vi "Process Data.vi"(8 "error in":errorcluster, 11 "Client Manager in":refnum<class "Client Manager.lvclass">) -> (0 "error out":errorcluster, 3 "Client Manager out":refnum<class "Client Manager.lvclass">)   [LabVIEW 2014, in "Client Manager.lvclass"]
uses:
  Client Manager.lvclass
  Topic Child Classes/Launch Client/Launch Client.lvclass
  Architecture/Classes/Topic_class/Topic.lvclass
panel:
  out "Client ID":string
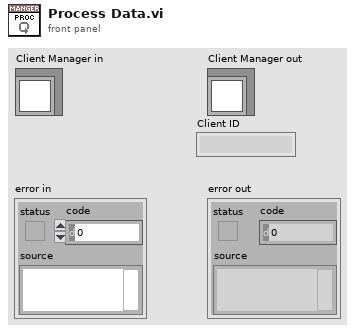
[diagram p1: front panel]
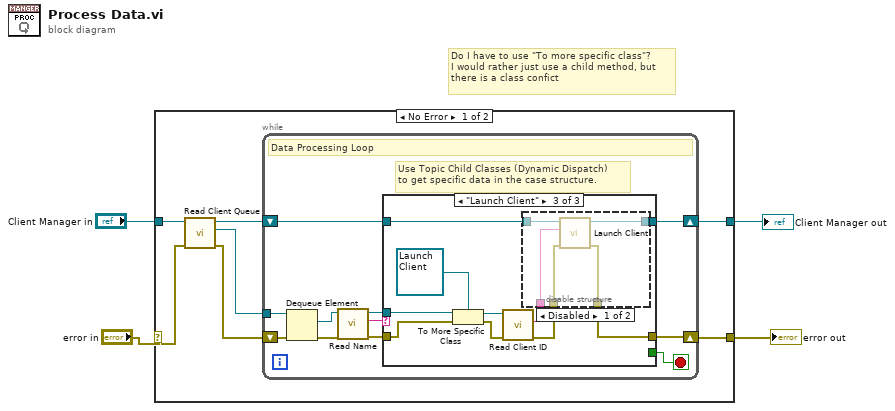
[diagram p0: block diagram]
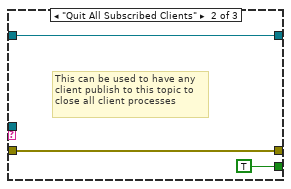
[diagram p3: hidden frame]
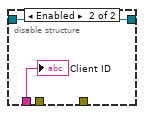
[diagram p4: hidden frame]
diagram:
  # "Do I have to use \"To more specific class\"?\nI would rather just use a child method, but\nthere is a class confict"
  n1 = case shown="No Error" "error in" {
    selector: "error in" -> [w5 w46]
    tunnel: [w6 w46] -> w2
    tunnel: [w8 w45] -> w3
    tunnel: "Client Manager in" -> [w11 w45]
    frame No Error {
      n2 = call-dynamic "Read Client Queue.vi"("error in"=w5, "Client in"=w11) -> ("error out"=w7:errorcluster, "Client Queue"=w10:refnum<queue>, "Client out"=w9:refnum<class "Client Manager.lvclass">)  [unwired: 7 in]
      n3 = while {
        tunnel: w10 -> [w22]
        shift-right: [w14] -> w8
        shift-left: w9 -> [w15]
        shift-right: [w12] -> w6
        shift-left: w7 -> [w13]
        stop <- w16 stop-if-true
        # "Use Topic Child Classes (Dynamic Dispatch)\nto get specific data in the case structure."
        # "Data Processing Loop"
        n4 = Dequeue Element(queue=w22, error in (no error)=w13) -> (element=w20:refnum<class "Topic.lvclass">, error out=w21:errorcluster)  [unwired: 1 in, 2 out]
        n5 = call-dynamic "Read Name.vi"("error in"=w21, "Topic in"=w20) -> ("error out"=w18:errorcluster, "Name"=w19:string, "Topic out"=w17:refnum<class "Topic.lvclass">)  [unwired: 7 in]
        n6 = case shown="\"Launch Client\"" w19 {
          tunnel: [_ TRUE _] -> w16
          tunnel: w18 -> [w24 w26 w32]
          tunnel: [w24 w26 w29] -> w12
          tunnel: w17 -> [_ _ w36]
          tunnel: w15 -> [w23 w25 w37]
          tunnel: [w23 w25 w28] -> w14
          frame Default {
          }
          frame "Quit All Subscribed Clients" {
            # "This can be used to have any\nclient publish to this topic to\nclose all client processes"
          }
          frame "Launch Client" {
            n7 = To More Specific Class(target class=refnum<class "Launch Client.lvclass"> refnum ("Launch Client.lvclass"), reference=w36, error in=w32) -> (specific class reference=w34:refnum<class "Launch Client.lvclass">, error out=w31:errorcluster)
            n8 = call-dynamic "Read Client ID.vi"("error in"=w31, "Launch Client in"=w34) -> ("error out"=w30:errorcluster, "Client ID"=w33:string)  [unwired: 7 in, 1 out]
            n9 = disable-structure shown="Disabled" {
              disable-tunnel: w37 -> [w42 w43]
              disable-tunnel: w33 -> [w41 w44]
              disable-tunnel: w30 -> [w39 _]
              disable-tunnel: [w38 _] -> w29
              disable-tunnel: [w40 w43] -> w28
              frame Disabled {
                n10 = call "Launch Client.vi"("error in"=w39, "Client Name"=w41, "Client Manager in"=w42) -> ("error out"=w38:errorcluster, "Client Manager out"=w40:refnum<class "Client Manager.lvclass">)  [unwired: 7 in]
              }
              frame Enabled {
                "Client ID" <- w44
              }
            }
          }
        }
      }
    }
    frame Error {
    }
  }
  "error out" <- w2
  "Client Manager out" <- w3
